vi "Read TCPStop.vi"(8 "error in (no error)":errorcluster, 11 "TCPController in":refnum<class "TCPController.lvclass">) -> (0 "error out":errorcluster, 2 "TCPStop":cluster{"Command":string, "Value":dbl}, 3 "TCPController out":refnum<class "TCPController.lvclass">)   [LabVIEW 2020, in "TCPController.lvclass"]
uses:
  TCPController.lvclass
  TCPController.lvclass/TCPController.ctl
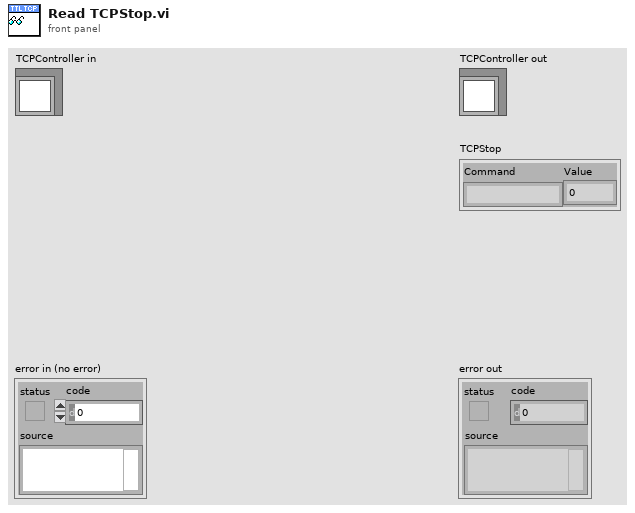
[diagram p1: front panel]
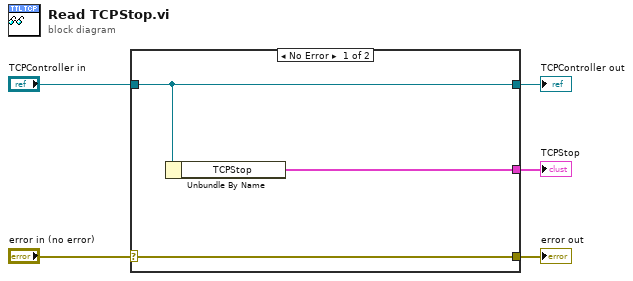
[diagram p0: block diagram]
diagram:
  n1 = case shown="No Error" "error in (no error)" {
    selector: "error in (no error)" -> [w8 w9]
    tunnel: [w8 w9] -> w4
    tunnel: [w7 w10] -> w2
    tunnel: "TCPController in" -> [w7 w10]
    tunnel: [w6 _] -> w1
    frame No Error {
      n2 = Unbundle By Name(w7) -> ("TCPStop"=w6:cluster{"Command":string, "Value":dbl})
    }
    frame Error {
    }
  }
  "error out" <- w4
  "TCPController out" <- w2
  "TCPStop" <- w1
